vi "mod.vi"(0 "number":u64, 1 "dzielnik":u64) -> (2 "reszta":u64, 3 "czesc calkowita":u64, 4 "czy 0?":bool)   [LabVIEW 2012]
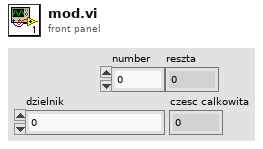
[diagram p1: front panel]
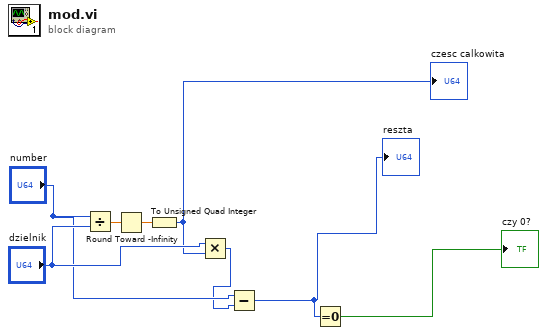
[diagram p0: block diagram]
diagram:
  n1 = Divide(x="number", y="dzielnik") -> (x/y=w7:ext)
  n2 = Round Toward -Infinity(1:w7) -> (0:w1:ext)
  n3 = To Unsigned Quad Integer(1:w1) -> (0:w5:u64)
  "czesc calkowita" <- w5
  n4 = Multiply(x="dzielnik", y=w5) -> (x*y=w3:u64)
  n5 = Subtract(x="number", y=w3) -> (x-y=w2:u64)
  "reszta" <- w2
  n6 = Equal To 0?(x=w2) -> (x = 0?=→"czy 0?":bool)
